vi "Dequeue.vi"(10 "Queue":refnum<data-value>) -> (0 "error out":errorcluster, 2 "Msg":refnum<class "Msg.lvclass">)   [LabVIEW 2021, in "jettl Queue Actor.lvlib"]
uses:
  Actor/Msg/Msg.lvclass
  jettl Queue Actor.lvlib
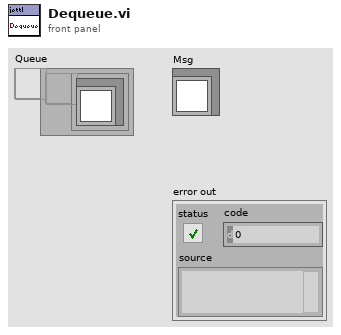
[diagram p1: front panel]
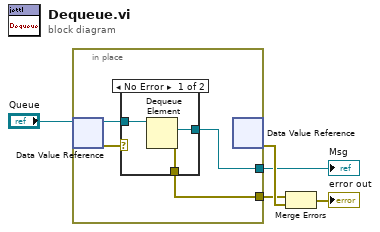
[diagram p0: block diagram]
diagram:
  n1 = in-place {
    in-place-border: [w8] -> w3
    in-place-border: [w7] -> w1
    n2 = in-place-dvr #1("Queue") -> (w9:refnum<queue>, w6:errorcluster)
    n3 = case shown="No Error" w6 {
      selector: w6 -> [_ w13]
      tunnel: w9 -> [w12 _]
      tunnel: [w11 w13] -> w8
      tunnel: [w10 _] -> w7
      frame No Error {
        n4 = Dequeue Element(queue=w12) -> (element=w10:refnum<class "Msg.lvclass">, error out=w11:errorcluster)  [unwired: 2 in, 2 out]
      }
      frame Error {
      }
    }
    n5 = in-place-dvr #1() -> (w4:errorcluster)  [unwired: 1 in, 1 out]
  }
  "Msg" <- w1
  n6 = Merge Errors(w3, w4) -> (→"error out":errorcluster)
